vi "OP Shield Config.vi"(8 "error in (no error)":errorcluster, 9 "Enum":enum16{"init", "Read", "Write"}(ring)=enum."Read", 10 "Shield in":u32, 11 "Path":path) -> (0 "error out":errorcluster, 1 "subarray":bool[](array[boolean]), 2 "Shield out":u32, 3 "Path out":path)   [LabVIEW 2014]
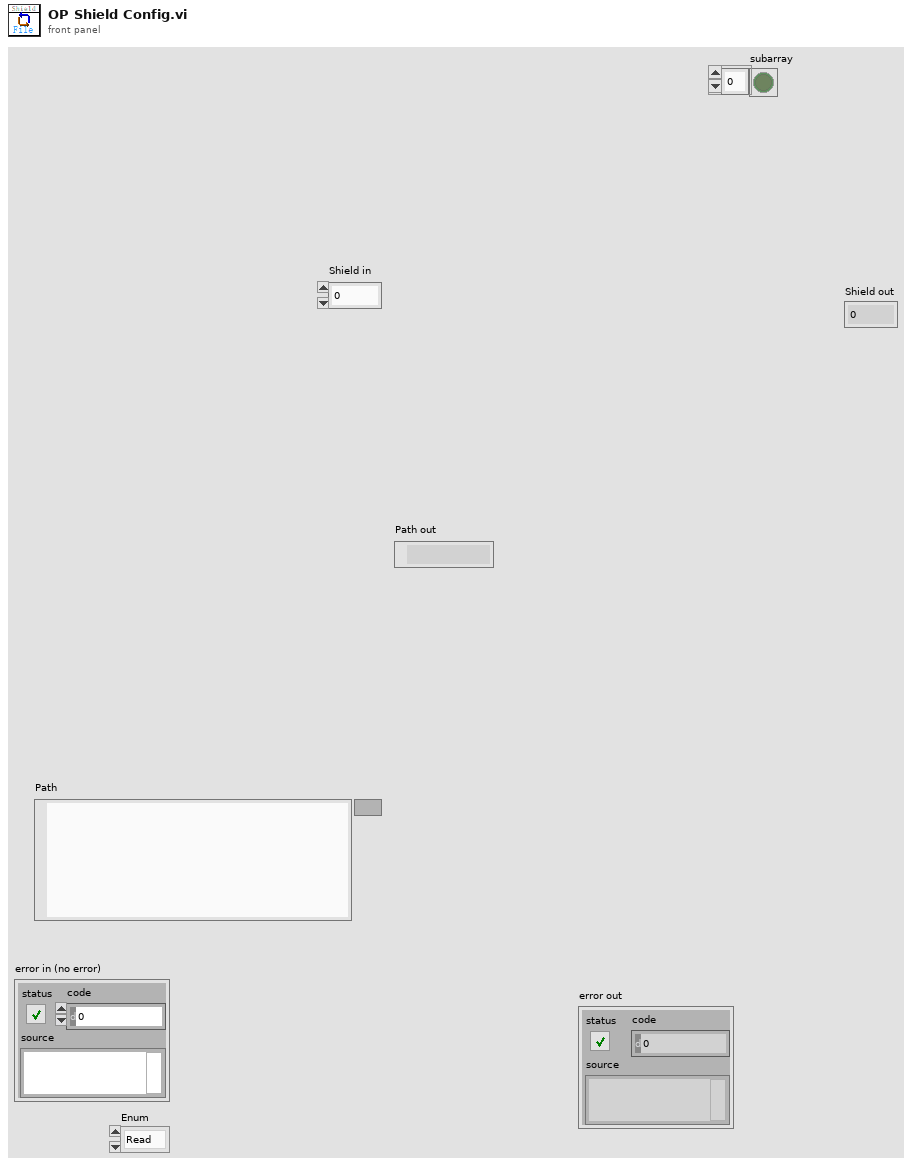
[diagram p1: front panel]
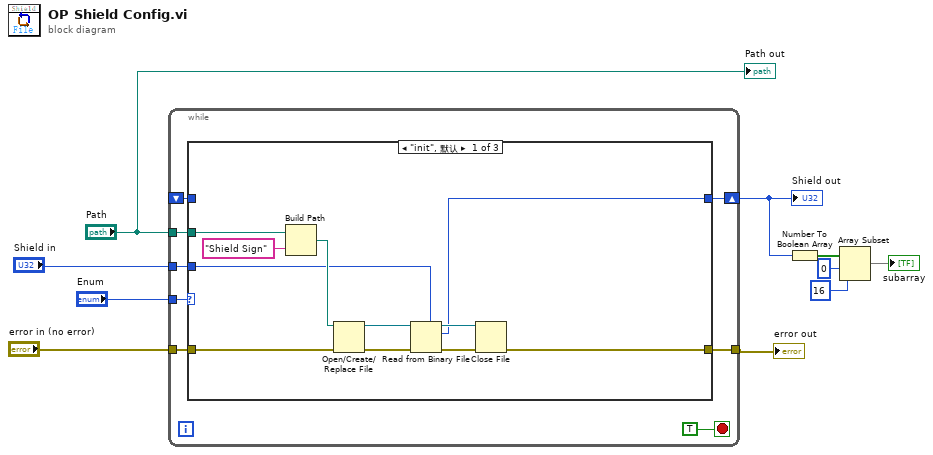
[diagram p0: block diagram]
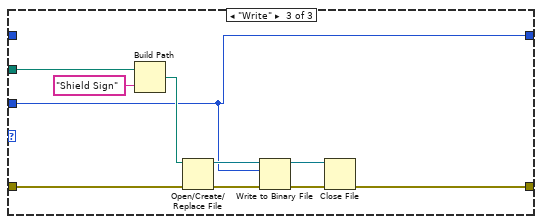
[diagram p3: hidden frame]
diagram:
  n1 = while {
    tunnel: "Enum" -> [w18]
    tunnel: "Path" -> [w17]
    tunnel: "error in (no error)" -> [w16]
    tunnel: "Shield in" -> [w15]
    shift-right: [w14] -> w5
    shift-left: _ -> [w12]
    tunnel: [w13] -> w7
    stop <- TRUE stop-if-true
    n2 = case shown="\"init\", 默认" w18 {
      tunnel: w17 -> [w28 _ w33]
      tunnel: w16 -> [w23 w30 w35]
      tunnel: w15 -> [w21 _ w32]
      tunnel: [w19 w31 w32] -> w14
      tunnel: [w20 w30 w34] -> w13
      tunnel: w12 -> [_ w31 _]
      frame "init", Default {
        n3 = Build Path(base path=w28, name or relative path="Shield Sign") -> (appended path=w22:path)
        n4 = Open/Create/Replace File(file path (use dialog)=w22, error in=w23) -> (refnum out=w27:refnum<file>, error out=w26:errorcluster)  [unwired: 4 in, 1 out]
        n5 = Read from Binary File(5:w21, 8:w26, 11:w27) -> (0:w24:errorcluster, 2:w19:u32, 3:w25:refnum<file>)  [unwired: 3 in, 1 out]
        n6 = Close File(refnum=w25, error in=w24) -> (error out=w20:errorcluster)  [unwired: 1 out]
      }
      frame "Read" {
      }
      frame "Write" {
        n7 = Build Path(base path=w33, name or relative path="Shield Sign") -> (appended path=w36:path)
        n8 = Open/Create/Replace File(file path (use dialog)=w36, error in=w35) -> (refnum out=w40:refnum<file>, error out=w39:errorcluster)  [unwired: 4 in, 1 out]
        n9 = Write to Binary File(file (use dialog)=w40, data=w32, error in=w39) -> (refnum out=w38:refnum<file>, error out=w37:errorcluster)  [unwired: 3 in, 1 out]
        n10 = Close File(refnum=w38, error in=w37) -> (error out=w34:errorcluster)  [unwired: 1 out]
      }
    }
  }
  "Shield out" <- w5
  "error out" <- w7
  n11 = Number To Boolean Array(number=w5) -> (Boolean array=w4:bool[])
  n12 = Array Subset(array=w4, index=0, length=16) -> (→"subarray":bool[])
  "Path out" <- "Path"
